vi "Init_available_Channels.vi"() -> (1 "AI.PhysicalChans":tag[](array[tag]))   [LabVIEW 2021]
uses:
  <resource>/objmgr/daqmx.rc
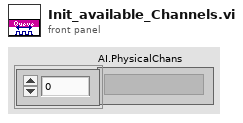
[diagram p1: front panel]
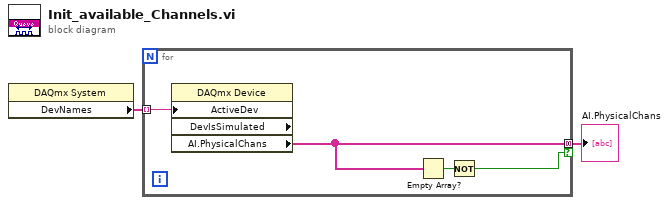
[diagram p0: block diagram]
diagram:
  n1 = property class="DAQmx System"() -> ("DevNames"=w1:tag[])  [unwired: 2 in, 2 out]
  n2 = for {
    tunnel: w1 -> [w6] mode=indexing
    tunnel: [w5] -> w2 mode=concatenating if=w3
    n3 = property class="DAQmx Device" props=["ActiveDev", "DevIsSimulated", "AI.PhysicalChans"]("ActiveDev"=w6) -> ("AI.PhysicalChans"=w5:tag[])  [unwired: 2 in, 3 out]
    n4 = Empty Array?(array=w5) -> (empty?=w4:bool)
    n5 = Not(x=w4) -> (.not. x?=w3:bool)
  }
  "AI.PhysicalChans" <- w2
